vi "threshold_write.vi"(4 "thresh_latch":bool, 5 "thresh_index":u8, 6 "thresh_f_ratio":u32, 7 "thresh_persistence":u32, 8 "thresh_new_max":fxp<+/-,32,16>, 9 "thresh_new_min":fxp<+/-,32,16>) -> ()   [LabVIEW 2018]
uses:
  <vilib>/rvi/DataTransferAndStorage/Container/XNode/niFpgaContainer.xnode
  <vilib>/rvi/Memory/Memory_Emulation/nirvimemoryEmulation.vi
  <vilib>/rvi/Memory/Memory_Emulation/nirvimemoryFastEmulation.vi
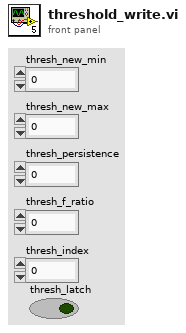
[diagram p1: front panel]
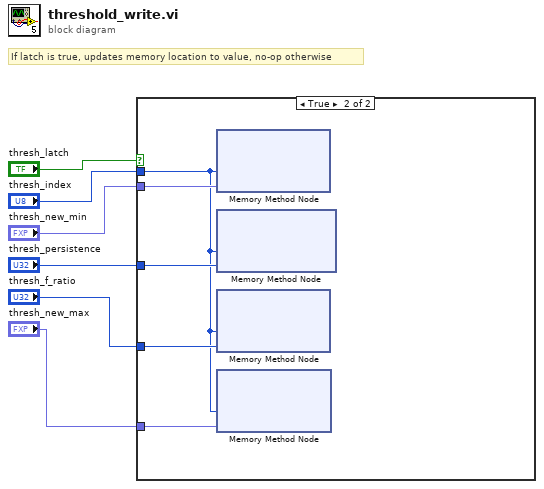
[diagram p0: block diagram]
diagram:
  # "If latch is true, updates memory location to value, no-op otherwise"
  n1 = case shown="True" "thresh_latch" {
    tunnel: "thresh_new_min" -> [_ w11]
    tunnel: "thresh_index" -> [_ w8]
    tunnel: "thresh_persistence" -> [_ w10]
    tunnel: "thresh_f_ratio" -> [_ w9]
    tunnel: "thresh_new_max" -> [_ w7]
    frame False {
    }
    frame True {
      n2 = xnode ("Memory Method Node")("Address"=w8, "Data"=w11) -> ()  [unwired: 1 in, 1 out]
      n3 = xnode ("Memory Method Node")("Address"=w8, "Data"=w10) -> ()  [unwired: 1 in, 1 out]
      n4 = xnode ("Memory Method Node")("Address"=w8, "Data"=w9) -> ()  [unwired: 1 in, 1 out]
      n5 = xnode ("Memory Method Node")("Address"=w8, "Data"=w7) -> ()  [unwired: 1 in, 1 out]
    }
  }
